vi "Dashboard Main.vi"() -> ()   [LabVIEW 2012]
uses:
  <vilib>/event_ctls.llb/eventvkey.ctl
  <vilib>/Utility/config.llb/NI_LVConfig.lvlib
  <vilib>/Utility/config.llb/Read Key (I32).vi
  <vilib>/Utility/config.llb/Write Key (I32).vi
  <vilib>/Utility/config.llb/Read Key (String).vi
  <vilib>/Utility/config.llb/Write Key (String).vi
  <vilib>/Rock Robotics/WPI/Camera/WPI_CameraFrameRate.ctl
  <vilib>/Rock Robotics/WPI/Camera/WPI_CameraExposure Values.ctl
  <vilib>/Rock Robotics/WPI/Camera/WPI_CameraWhite Balance Values.ctl
  <vilib>/Rock Robotics/WPI/Camera/WPI_CameraImageSize.ctl
panel:
  in  "Image Size":T1=enum."160x120"
  in  "Camera?":bool
  out "Battery Value":dbl(slide) scale=0.0..14.0 scale format="%#_2e"
  out "Battery":sgl(graph)
  in  "Camera Settings":T2={"Frate Rate"=30, "Compression"=30, "Size"=1} {"Frate Rate" scale=1.0..30.0; "Size" items=["640x480", "320x240", "160x120"]}
  out "Mode":T3(ring)=enum."Auto Disabled"
  out "Camera IP":string
  out "JS1 Z":dbl(slide) scale=-1.0..1.0 scale format="%#_2e"
  out "JS2 Z":dbl(slide) scale=-1.0..1.0 scale format="%#_2e"
  out "Joystick 1":cluster{"X":dbl, "Y":dbl}[](graph)
  out "Joystick 2":cluster{"X":dbl, "Y":dbl}[](graph)
  out "JS Buttons 1":T4
  out "JS Buttons 2":T4
  out "MotorSlide4":dbl(slide) scale=-1.0..1.0 scale format="%#_2e"
  out "MotorSlide3":dbl(slide) scale=-1.0..1.0 scale format="%#_2e"
  out "MotorSlide2":dbl(slide) scale=-1.0..1.0 scale format="%#_2e"
  in  "MotorName3":string="Front Left"
  in  "MotorName4":string="Front Right"
  in  "MotorName1":string="Rear Left"
  in  "MotorName2":string="Rear Right"
  out "MotorChart4":dbl(graph)
  out "MotorChart3":dbl(graph)
  out "MotorChart2":dbl(graph)
  out "MotorSlide1":dbl(slide) scale=-1.0..1.0 scale format="%#_2e"
  out "MotorChart1":dbl(graph)
  out "Robot IP":string
  in  "Dashboard Tab":enum32{"Operation", "Test", "Checklist"}(tab)
  in  "Checkbox 2":bool
  in  "Checkbox 1":bool
  in  "Slider 1":dbl(slide) scale=0.0..100.0
  in  "Slider":dbl(slide) scale=0.0..100.0 scale format="%#_3g"
  in  "On/Off":bool caption="Solenoid"
  in  "Test Name":u16(ring) items=["Select the test to run...", "Example Test", "-------------------------------", "List of tests is built in robot code.", "Replace with your own automated tests."]
  in  "Test Tree":string(tree)
  in  "Motor":cluster{"Value":dbl, "Enable":bool} {"Value" scale=-1.0..1.0 scale format="%#_3g"}
  out "Progress":T5 {"Test Progress" scale=0.0..100.0}
  in  "Rev/Fwd":cluster{"Forward":bool, "Reverse":bool}
  in  "Ring":u16(ring) items=["Auto", "Fixed indoor", "Fixed outdoor 1", "Fixed outdoor 2", "Fixed fluorescent 1", "Fixed fluorescent 2", "Hold current"]
  in  "Listbox":i32(listbox)
  in  "Viewer":T6(tab)
  out "Mbps":dbl format="%#.1g"
  in  "Enable":bool
  in  "DB Camera Config":bool
  out "Mbps":bool
  out "fps":dbl format="%#.1g"
  out "Image Error Message":string="Timeout in Camera Communications"
  out "Camera Image":T7(plugin-control)
  out "Tree":string(tree)
  # "Drive & Motors"
  # "Robot IP:"
  # "Customize by placing controls and indicators here and name to match\nDashboard Variables on robot."
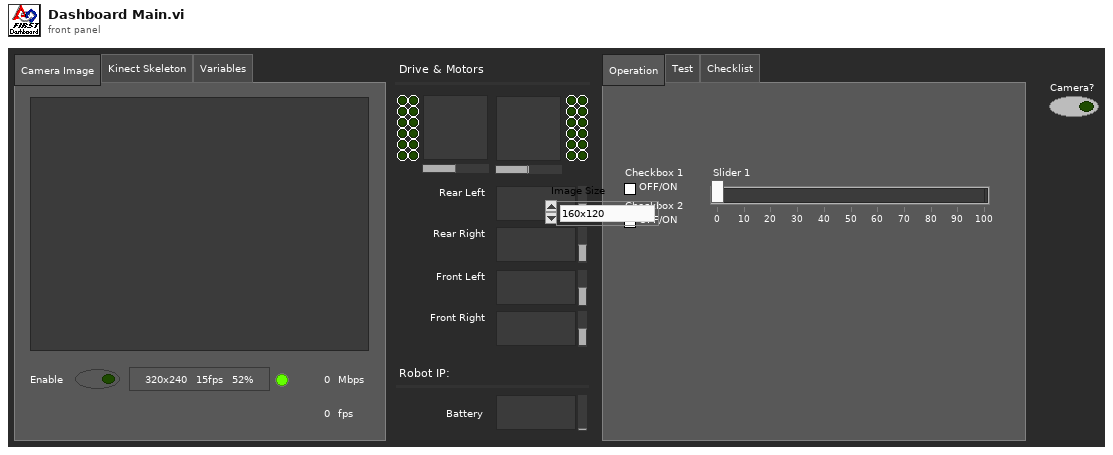
[diagram p1: front panel]
types:
  T1 = typedef "WPI_CameraImageSize.ctl" = enum16{"640x480", "320x240", "160x120"}
  T2 = cluster{"Frate Rate":i32, "Compression":i32, "Size":u16}
  T3 = enum8{"Tele-Op Disabled", "Tele-Op Enabled", "Auto Disabled", "Auto Enabled", "Test Disabled", "Test Enabled", ""}
  T4 = cluster{bool, bool, bool, bool, bool, bool, bool, bool, bool, bool, bool, bool}
  T5 = cluster{"Test Progress":u8, "Test Progress Text":string}
  T6 = enum32{"Camera Image", "Kinect Skeleton", "Variables"}
  T7 = typedef "IMAQ Image.ctl" = refnum<image>
  T8 = typedef "Image Type" = u32
  T9 = typedef "LVRectTypeDef.ctl" = cluster{"Left":i16, "Top":i16, "Right":i16, "Bottom":i16}
  T10 = typedef "WPI_CameraFrameRate.ctl" = u32
  T11 = typedef "WPI_CameraExposure Values.ctl" = enum16{"Auto", "Flicker-free 50 Hz", "Flicker-free 60 Hz", "Hold current"}
  T12 = typedef "WPI_CameraWhite Balance Values.ctl" = enum16{"Auto", "Fixed indoor", "Fixed outdoor 1", "Fixed outdoor 2", "Fixed fluorescent 1", "Fixed fluorescent 2", "Hold current"}
  T13 = typedef "WPI_CameraDevRef.ctl" = cluster{"Camera Address":string, "CameraStatus":errorcluster, "Acquire Image Notifier":refnum<notifier>}
  T14 = cluster{"Competition mode":bool, "Robot Link":bool, "Autonomous":bool, "Enabled":bool, "E-Stop":bool, "Simulated":bool, "TestMode":bool, "Docked Window":bool}
  T15 = cluster{"Boolean Array[0]":bool, "Boolean Array[1]":bool, "Boolean Array[2]":bool, "Boolean Array[3]":bool, "Boolean Array[4]":bool, "Boolean Array[5]":bool, "Boolean Array[6]":bool, "Boolean Array[7]":bool, "Boolean Array[8]":bool, "Boolean Array[9]":bool, "Boolean Array[10]":bool, "Boolean Array[11]":bool}
  T16 = typedef "NI_LVConfig.lvlib/Config Data RefNum.ctl" = refnum<k1>
  T17 = typedef "eventvkey.ctl" = enum16{"ASCII", "Enter", "Return", "Shift", "Ctrl", "Alt", "Cmd", "Opt", "Caps", "NumLock", "Clear", "Break", "Up", "Down", "Left", "Right", "Insert", "Delete", "Home", "End", "PageUp", "PageDown", "Escape", "Help", "Pause", "ScrollLock", "F1", "F2", "F3", "F4", "F5", "F6", "F7", "F8", "F9", "F10", "F11", "F12", "F13", "F14", "F15", "F16", "F17", "F18", "F19", "F20", "F21", "F22", "F23", "F24", "Play", "VolumeUp", "VolumeDown", "Mute", "Two Byte Char"}
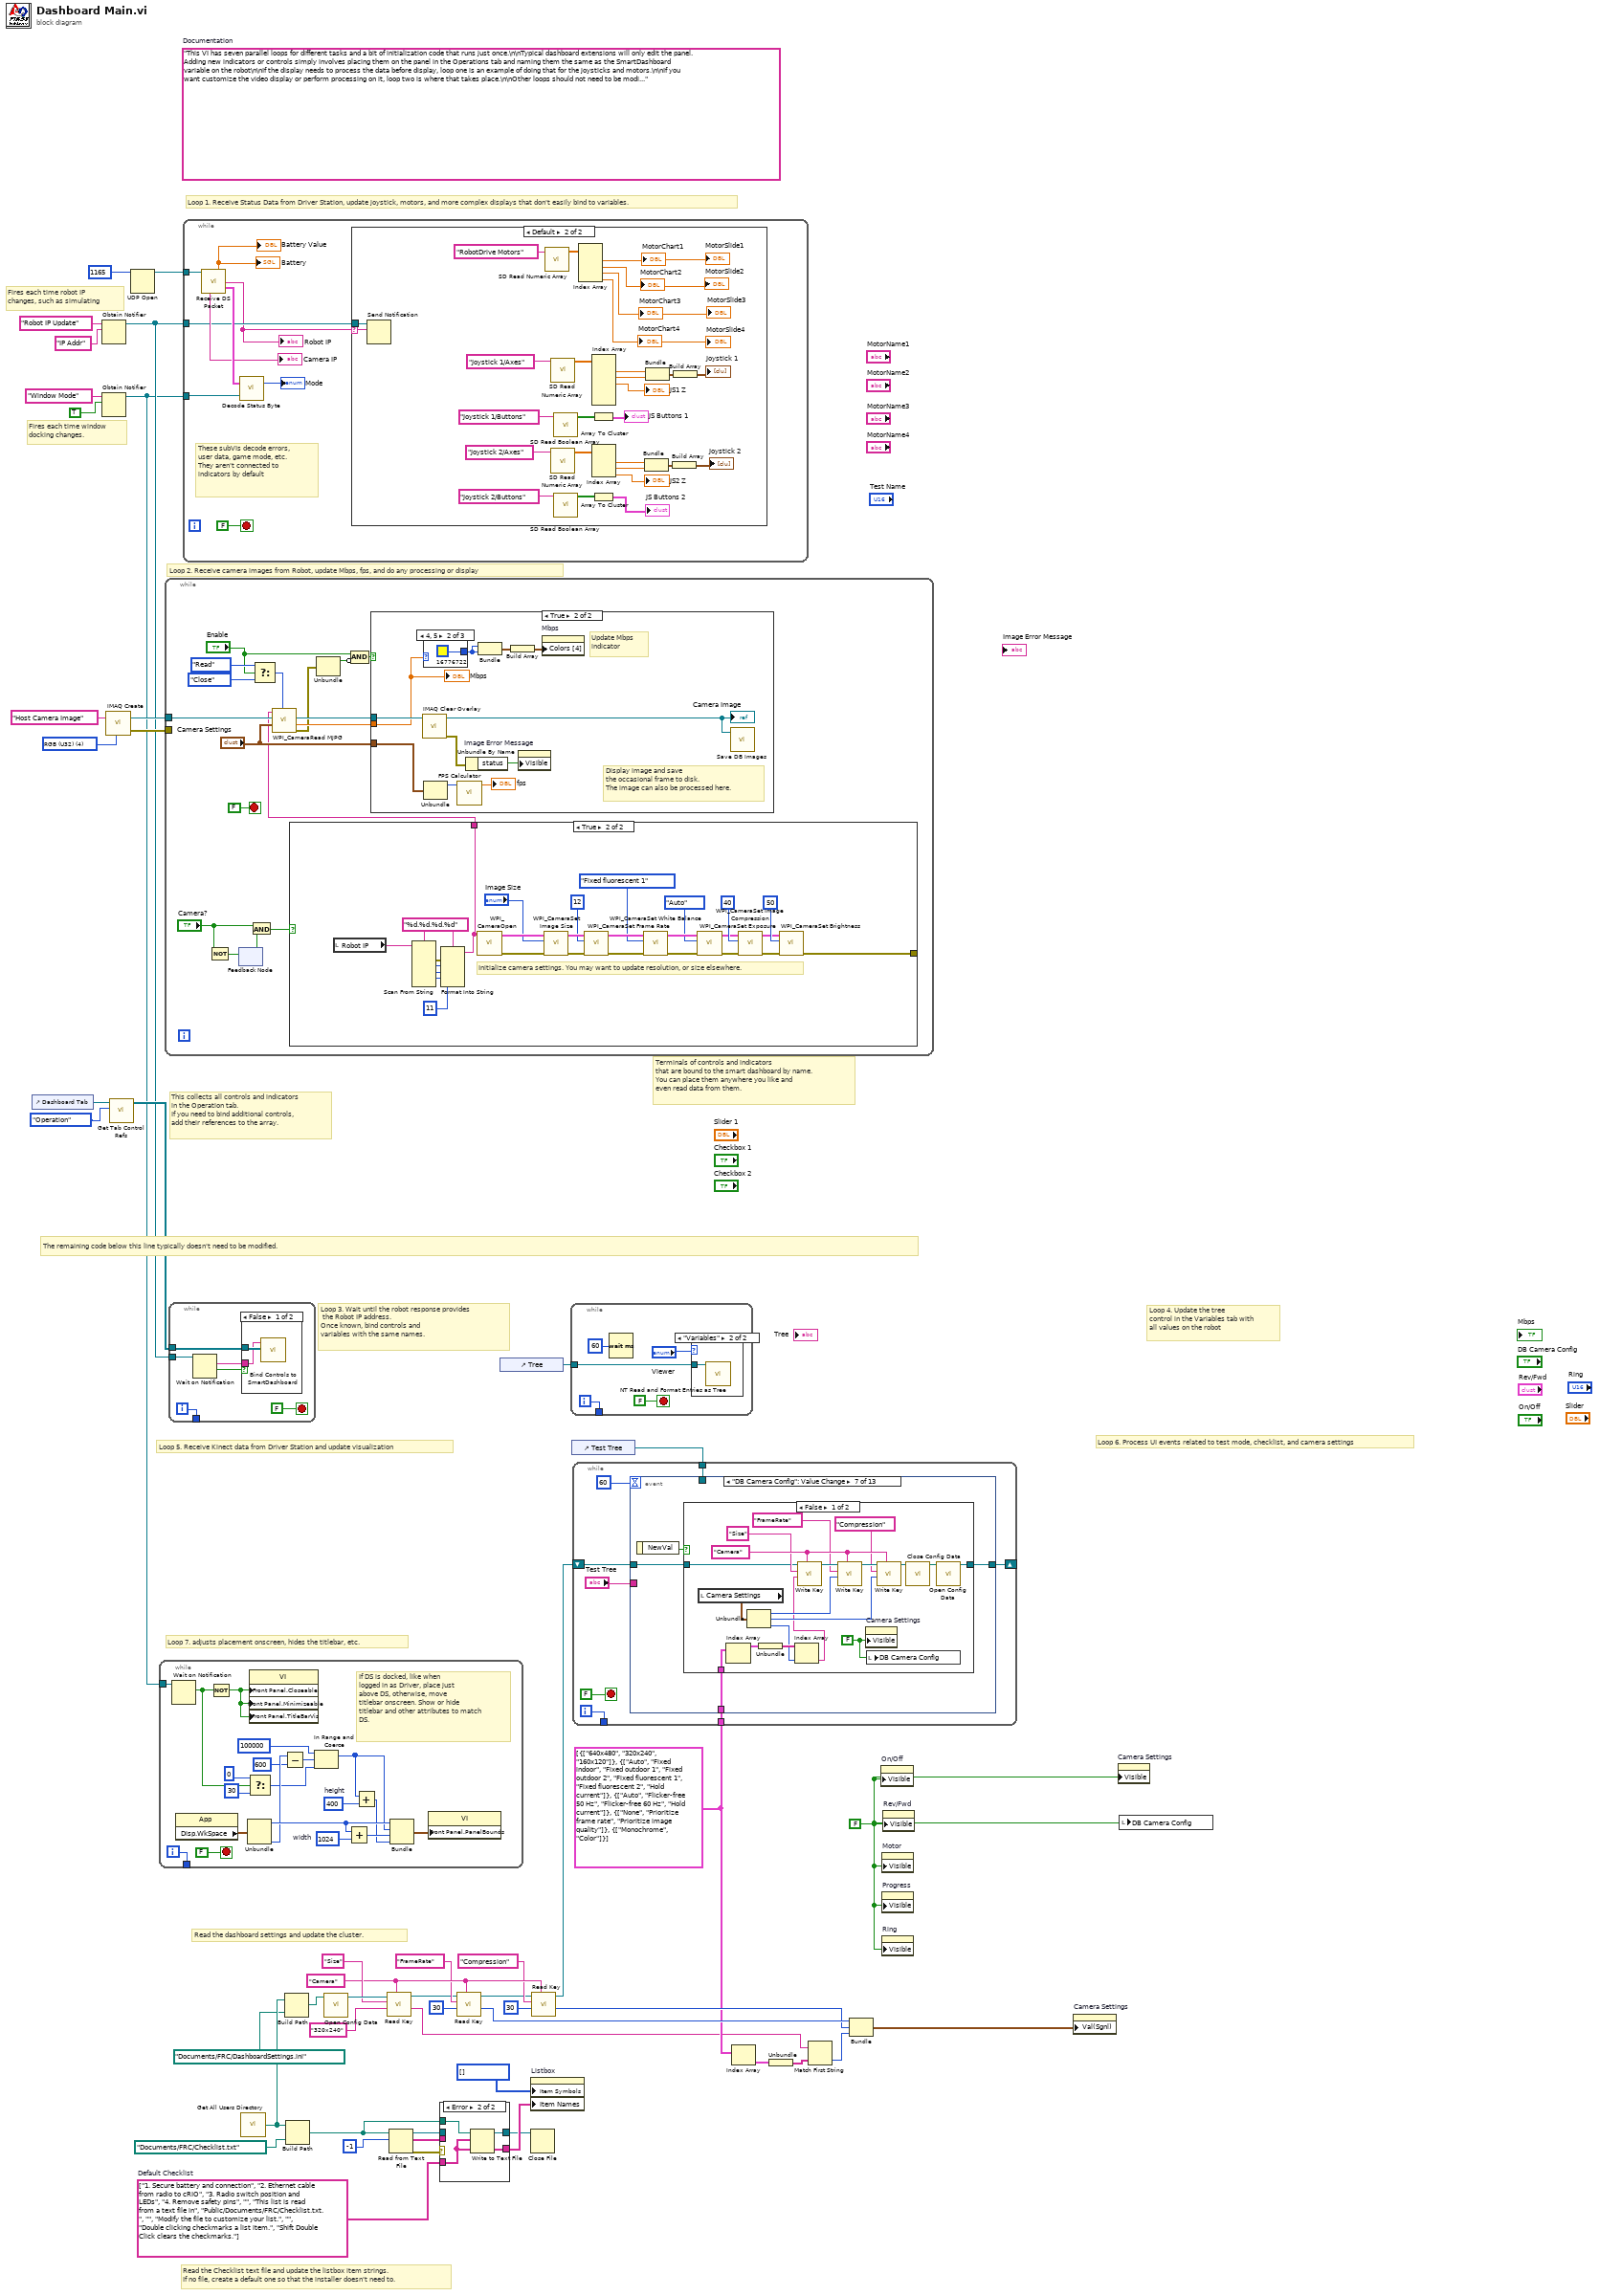
[diagram p0: block diagram]
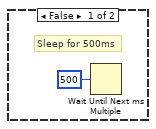
[diagram p4: hidden frame]
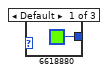
[diagram p5: hidden frame]
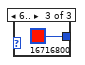
[diagram p6: hidden frame]
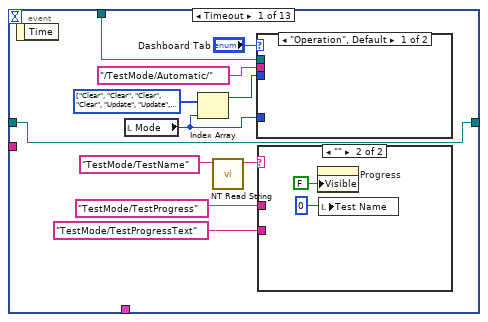
[diagram p8: hidden frame]
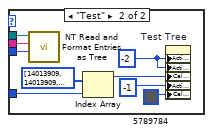
[diagram p9: hidden frame]
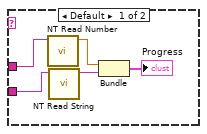
[diagram p10: hidden frame]
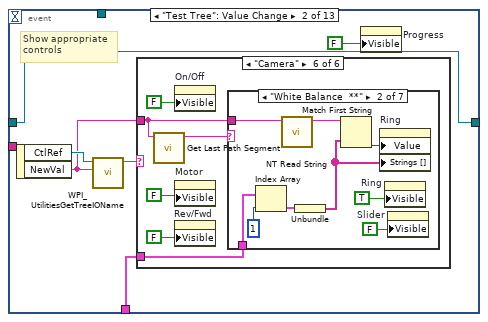
[diagram p11: hidden frame]
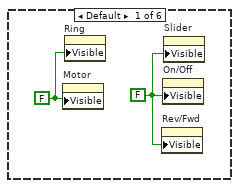
[diagram p12: hidden frame]
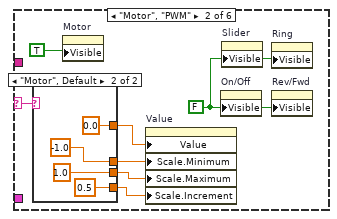
[diagram p13: hidden frame]
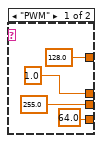
[diagram p14: hidden frame]
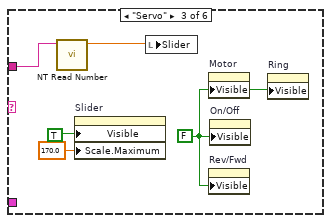
[diagram p15: hidden frame]
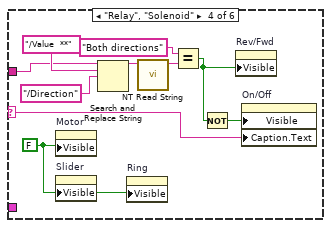
[diagram p16: hidden frame]
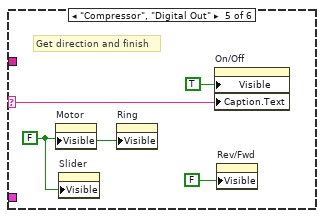
[diagram p17: hidden frame]
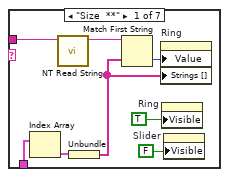
[diagram p18: hidden frame]
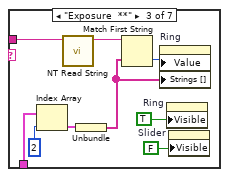
[diagram p19: hidden frame]
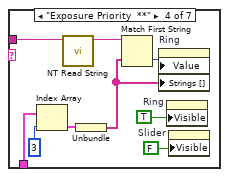
[diagram p20: hidden frame]
diagram:
  w21 = "Camera"
  w13 = cluster{string[]}[] [{["640x480", "320x240", "160x120"]}, {["Auto", "Fixed indoor", "Fixed outdoor 1", "Fixed outdoor 2", "Fixed fluorescent 1", "Fixed fluorescent 2", "Hold current"]}, {["Auto", "Flicker-free 50 Hz", "Flicker-free 60 Hz", "Hold current"]}, {["None", "Prioritize frame rate", "Prioritize image quality"]}, {["Monochrome", "Color"]}]
  w29 = string[] ["1. Secure battery and connection", "2. Ethernet cable from radio to cRIO", "3. Radio switch position and LEDs", "4. Remove safety pins", "", "This list is read from a text file in", "Public/Documents/FRC/Checklist.txt.", "", "Modify the file to customize your list.", "", "Double clicking checkmarks a list item.", "Shift Double Click clears the checkmarks."]  # Default Checklist
  w27 = FALSE ("Visible")
  (unwired) "This VI has seven parallel loops for different tasks and a bit of initialization code that runs just once.\n\nTypical dashboard extensions will only edit the panel. Adding new indicators or controls simply involves placing them on the panel in the Operations tab and naming them the same as the SmartDashboard variable on the robot\n\nIf the display needs to process the data before display, loop one is an example of doing that for the joysticks and motors.\n\nIf you want customize the video display or perform processing on it, loop two is where that takes place.\n\nOther loops should not need to be modified. They are pretty standard, and document the task they perform."  # Documentation
  w48 = T8 4 items=["Grayscale (U8)", "Grayscale (I16)", "Grayscale (SGL)", "Complex (CSG)", "RGB (U32)", "HSL (U32)", "RGB (U64)"] ("Image Type")
  # "Fires each time robot IP\nchanges, such as simulating"
  # "Fires each time window\ndocking changes."
  # "Read the Checklist text file and update the listbox item strings.\nIf no file, create a default one so that the installer doesn't need to."
  # "This collects all controls and indicators\nin the Operation tab.\nIf you need to bind additional controls,\nadd their references to the array."
  # "The remaining code below this line typically doesn't need to be modified."
  # "Loop 6. Process UI events related to test mode, checklist, and camera settings"
  # "Read the dashboard settings and update the cluster."
  # "Terminals of controls and indicators\nthat are bound to the smart dashboard by name.\nYou can place them anywhere you like and\neven read data from them."
  # "Loop 4. Update the tree\ncontrol in the Variables tab with\nall values on the robot"
  # "Loop 3. Wait until the robot response provides\n the Robot IP address.\nOnce known, bind controls and\nvariables with the same names."
  # "Loop 5. Receive Kinect data from Driver Station and update visualization"
  # "Loop 7. adjusts placement onscreen, hides the titlebar, etc."
  # "Loop 1. Receive Status Data from Driver Station, update joystick, motors, and more complex displays that don't easily bind to variables."
  # "Loop 2. Receive camera images from Robot, update Mbps, fps, and do any processing or display"
  n1 = control-ref of="Dashboard Tab"() -> (w43:refnum<vi>)
  n2 = Obtain Notifier(name (unnamed)="Robot IP Update", notification data type="IP Addr" ("name (unnamed)")) -> (notifier out=w40:refnum<notifier>)  [unwired: 2 in, 2 out]
  n3 = Obtain Notifier(name (unnamed)="Window Mode", notification data type=TRUE) -> (notifier out=w33:refnum<notifier>)  [unwired: 2 in, 2 out]
  n4 = call "IMAQ Create"("Image Name"="Host Camera Image", "Image Type"=w48) -> ("New Image"=w46:T7, "error out"=w45:errorcluster)  [unwired: 2 in, 1 out]
  n5 = call <vilib>:"Get Tab Control Refs.vi"("Page Index"=enum32{"Operation", "Test"}."Operation" ("Dashboard Tab"), "TabControl in"=w43) -> ("ControlsOnPage"=w44:refnum<vi>[])  [unwired: 9 in]
  n6 = UDP Open(11:u16 1165 ("port")) -> (port=w49:refnum<k16>)  [unwired: 2 in, 4 out]
  n7 = while {
    tunnel: w33 -> [w69]
    tunnel: [w67] -> _
    i -> [w67]
    stop <- FALSE stop-if-true
    w59 = 1024  # width
    w62 = 400  # height
    # "If DS is docked, like when\nlogged in as Driver, place just\nabove DS, otherwise, move\ntitlebar onscreen. Show or hide\ntitlebar and other attributes to match\nDS."
    n8 = Wait on Notification(notifier=w69) -> (notification=w54:bool)  [unwired: 3 in, 3 out]
    n9 = property class="App"() -> ("Disp.WkSpace"=w65:T9)  [unwired: 2 in, 2 out]
    n10 = Not(x=w54) -> (.not. x?=w68:bool)
    n11 = Unbundle(w65) -> ("Left"=w63:i16, "Bottom"=w60:i16)  [unwired: 2 out]
    n12 = Select(t=0, s=w54, f=30) -> (s? t:f=w53:i32)
    n13 = property class="VI"("Front Panel.Closeable"=w68, "Front Panel.Minimizeable"=w68, "Front Panel.TitleBarVis"=w68) -> ()  [unwired: 2 in, 2 out]
    n14 = Subtract(x=w60, y=600) -> (x-y=w57:i32)
    n15 = In Range and Coerce(upper limit=100000, x=w57, lower limit=w53) -> (coerced(x)=w51:i32)  [unwired: 1 out]
    n16 = Add(x=w63, y=w59) -> (x+y=w64:i32)
    n17 = Add(x=w51, y=w62) -> (x+y=w61:i32)
    n18 = Bundle("Left"=w63, w51, w64, w61) -> (w66:cluster{"Left":i16, i32, i32, i32})  [unwired: 1 out]
    n19 = property class="VI"("Front Panel.PanelBounds"=w66) -> ()  [unwired: 2 in, 2 out]
  }
  n20 = while {
    tunnel: w46 -> [w85]
    tunnel: w45 -> [_]
    stop <- FALSE stop-if-true
    n21 = Not(x="Camera?") -> (.not. x?=w75:bool)
    n22 = feedback #1() -> (w74:bool)  [unwired: 1 in]
    n23 = feedback-in #1(w75) -> ()
    n24 = And(x="Camera?", y=w74) -> (x .and. y?=w72:bool)
    n25 = Select(t=enum16{"Read", "Reopen", "Close"}."Read" ("Operation"), s="Enable", f=enum16{"Read", "Reopen", "Close"}."Close" ("Operation")) -> (s? t:f=w80:enum16{"Read", "Reopen", "Close"})
    n26 = case shown="True" w72 {
      tunnel: [_ w89] -> _
      tunnel: [_ w88] -> w71
      frame False {
      }
      frame True {
        w96 = "%d.%d.%d.%d" ("format string")
        # "Initialize camera settings. You may want to update resolution, or size elsewhere."
        n27 = local read "Robot IP"() -> (w90:string)
        n28 = Scan From String(format string=w96, input string=w90) -> (error out=w94:errorcluster, output 1=w93:i32, output 2=w92:i32, output 3=w91:i32)  [unwired: 2 in, 7 out]
        n29 = Format Into String(format string=w96, error in=w94, w93, w92, w91, 11 ("IP Suffix:")) -> (resulting string=w88:string)  [unwired: 1 in, 1 out]
        n30 = call <vilib>:"WPI_CameraOpen.vi"("Camera Address"=w88) -> ("error out"=w106:errorcluster, "CameraDevRef"=w107:T13)  [unwired: 2 in, 7 out]
        n31 = call <vilib>:"WPI_CameraSet Image Size.vi"("error in (no error)"=w106, "Image Size"="Image Size", "CameraDevRef"=w107) -> ("error out"=w105:errorcluster, "CameraDevRef Out"=w108:T13)  [unwired: 7 out]
        n32 = call <vilib>:"WPI_CameraSet Frame Rate.vi"("error in (no error)"=w105, "Frame Rate (fps)"=T10 12, "CameraDevRef"=w108) -> ("error out"=w104:errorcluster, "CameraDevRef Out"=w110:T13)  [unwired: 7 out]
        n33 = call <vilib>:"WPI_CameraSet White Balance.vi"("error in (no error)"=w104, "White Balance"=WPI_CameraWhite_Balance_Values."Fixed fluorescent 1", "CameraDevRef"=w110) -> ("error out"=w103:errorcluster, "CameraDevRef Out"=w109:T13)  [unwired: 7 out]
        n34 = call <vilib>:"WPI_CameraSet Exposure.vi"("error in (no error)"=w103, "Exposure"=WPI_CameraExposure_Values."Auto", "CameraDevRef"=w109) -> ("error out"=w102:errorcluster, "CameraDevRef Out"=w112:T13)  [unwired: 7 out]
        n35 = call <vilib>:"WPI_CameraSet Image Compression.vi"("error in (no error)"=w102, "Compression"=40, "CameraDevRef"=w112) -> ("error out"=w101:errorcluster, "CameraDevRef Out"=w111:T13)  [unwired: 7 out]
        n36 = call <vilib>:"WPI_CameraSet Brightness.vi"("error in (no error)"=w101, "Brightness"=50, "CameraDevRef"=w111) -> ("error out"=w89:errorcluster)  [unwired: 8 out]
      }
    }
    n37 = call <vilib>:"WPI_CameraRead MJPG.vi"("Operation"=w80, "Camera Settings"="Camera Settings", "Image"=w85, "address"=w71) -> ("error out"=w79:errorcluster, "Bandwidth (kbps)"=w83:dbl, "Image Out"=w84:T7)  [unwired: 5 in]
    n38 = Unbundle(w79) -> ("status"=w77:bool)  [unwired: 2 out]
    n39 = Compound Arithmetic op=AND("Enable", invert w77) -> (w76:bool)
    n40 = case shown="True" w76 {
      tunnel: "Camera Settings" -> [_ w117]
      tunnel: w84 -> [_ w120]
      tunnel: w83 -> [_ w119]
      frame False {
        # "Sleep for 500ms"
        n41 = Wait Until Next ms Multiple(millisecond multiple=u32 500) -> ()  [unwired: 1 out]
      }
      frame True {
        # "Display image and save\nthe occasional frame to disk.\nThe image can also be processed here."
        # "Update Mbps\nindicator"
        n42 = call "IMAQ Clear Overlay"("Image"=w120) -> ("error out"=w125:errorcluster, "Image Out"=w124:T7)  [unwired: 2 in, 7 out]
        "Camera Image" <- w124
        n43 = case shown="4, 5" w119 {
          tunnel: [u32 6618880 ("Color Box") u32 16776722 ("Color Box") u32 16716800 ("Color Box")] -> w121
          frame Default {
          }
          frame 4, 5 {
          }
          frame 6.. {
          }
        }
        n44 = Unbundle(w117) -> ("Frate Rate"=w116:i32)  [unwired: 2 out]
        n45 = call "FPS Calculator.vi"("Average Count"=w116) -> ("fps"=→"fps":dbl)  [unwired: 10 in]
        n46 = Unbundle By Name(w125) -> ("status"=w126:bool)
        n47 = Bundle("Color Box"=w121, "Color Box"=w121) -> (w123:cluster{"Color Box":u32, "Color Box":u32})  [unwired: 1 out]
        n48 = Build Array(w123) -> (w122:cluster{"Color Box":u32, "Color Box":u32}[])
        n49 = property on="Image Error Message" class="Str"("Visible"=w126) -> ()  [unwired: 2 in, 2 out]
        n50 = property on="Mbps" class="Bool (strict)"("Colors [4]"=w122) -> ()  [unwired: 2 in, 2 out]
        n51 = call "Save DB Images.vi"("Image"=w124) -> ()  [unwired: 2 in, 1 out]
        "Mbps" <- w119
      }
    }
  }
  n52 = while {
    tunnel: w44 -> [w135]
    tunnel: w40 -> [w132]
    tunnel: [w130] -> _
    i -> [w130]
    stop <- FALSE stop-if-true
    n53 = Wait on Notification(notifier=w132) -> (notification=w131:string, timed out?=w133:bool)  [unwired: 3 in, 2 out]
    n54 = case shown="False" w133 {
      tunnel: w135 -> [w137 _]
      tunnel: w131 -> [w136 _]
      frame False {
        n55 = call <vilib>:"Bind Controls to SmartDashboard.vi"("Bound Control Refs"=w137, "Server IP Address"=w136) -> ()  [unwired: 10 in]
      }
      frame True {
      }
    }
  }
  n56 = while {
    tunnel: w49 -> [w144]
    tunnel: w40 -> [w139]
    tunnel: w33 -> [w142]
    stop <- FALSE stop-if-true
    # "These subVIs decode errors, user data, game mode, etc.\nThey aren't connected to indicators by default"
    n57 = call "Receive DS Packet.vi"("Recv Socket"=w144) -> ("Battery"=→"Battery" →"Battery Value":sgl, "Robot IP Address"=w138:string, "Status"=w145:T14, "Camera IP Address"=→"Camera IP":string)  [unwired: 1 in, 10 out]
    "Robot IP" <- w138
    n58 = call "Decode Status Byte.vi"("Window Mode Notifier"=w142, "Status"=w145) -> ("Mode"=→"Mode":T3)  [unwired: 1 out]
    n59 = case shown="Default" w138 {
      selector: w138 -> [_ w147]
      tunnel: w139 -> [_ w148]
      frame "0.0.0.0" {
        # "Robot not responding, don't poll the variables"
      }
      frame Default {
        n60 = Send Notification(notification=w147, notifier=w148) -> ()  [unwired: 1 in, 2 out]
        n61 = call <vilib>:"SD Read Numeric Array.vi"("Name"="RobotDrive Motors") -> ("Numeric Array"=w171:dbl[])  [unwired: 8 in, 2 out]
        n62 = call <vilib>:"SD Read Numeric Array.vi"("Name"="Joystick 1/Axes") -> ("Numeric Array"=w164:dbl[])  [unwired: 8 in, 2 out]
        n63 = call <vilib>:"SD Read Numeric Array.vi"("Name"="Joystick 2/Axes") -> ("Numeric Array"=w158:dbl[])  [unwired: 8 in, 2 out]
        n64 = call <vilib>:"SD Read Boolean Array.vi"("Name"="Joystick 1/Buttons") -> ("Boolean Array"=w166:bool[])  [unwired: 8 in, 2 out]
        n65 = call <vilib>:"SD Read Boolean Array.vi"("Name"="Joystick 2/Buttons") -> ("Boolean Array"=w157:bool[])  [unwired: 8 in, 2 out]
        n66 = Index Array(array=w171) -> (element #1=→"MotorChart1" →"MotorSlide1":dbl, element #2=→"MotorSlide2" →"MotorChart2":dbl, element #3=→"MotorChart3" →"MotorSlide3":dbl, element #4=→"MotorChart4" →"MotorSlide4":dbl)  [unwired: 4 in]
        n67 = Array To Cluster(array=w166) -> (cluster=→"JS Buttons 1":T15)
        n68 = Array To Cluster(array=w157) -> (cluster=→"JS Buttons 2":T15)
        n69 = Index Array(array=w164) -> (element #1=w161:dbl, element #2=w162:dbl, element #3=→"JS1 Z":dbl)  [unwired: 6 in, 3 out]
        n70 = Index Array(array=w158) -> (element #1=w153:dbl, element #2=w152:dbl, element #3=→"JS2 Z":dbl)  [unwired: 3 in]
        n71 = Bundle("Numeric"=w153, "Numeric"=w152) -> (w154:cluster{"Numeric":dbl, "Numeric":dbl})  [unwired: 1 in]
        n72 = Bundle("Numeric"=w161, "Numeric"=w162) -> (w160:cluster{"Numeric":dbl, "Numeric":dbl})  [unwired: 1 in]
        n73 = Build Array(w154) -> (→"Joystick 2":cluster{"Numeric":dbl, "Numeric":dbl}[])
        n74 = Build Array(w160) -> (→"Joystick 1":cluster{"Numeric":dbl, "Numeric":dbl}[])
      }
    }
  }
  n75 = call "Get All Users Directory.vi"() -> ("All User Path"=w26:path)
  n76 = Build Path(base path=w26, name or relative path=path "Documents/FRC/DashboardSettings.ini") -> (appended path=w25:path)
  n77 = Build Path(base path=w26, name or relative path=path "Documents/FRC/Checklist.txt") -> (appended path=w30:path)
  n78 = call <vilib>:"Open Config Data.vi"("configuration file path"=w25) -> ("refnum"=w24:T16)  [unwired: 8 in, 2 out]
  n79 = call-poly <vilib>:"Read Key.vi"("section"=w21, "default value"="320x240", "key"="Size", "refnum"=w24) -> ("value"=w11:string, "refnum out"=w6:T16)  [unwired: 2 in, 4 out]
  n80 = Read from Text File(file (use dialog)=w30, count=-1 ("timeout ms (25000)")) -> (refnum out=w8:refnum<file>, text=w31:string[], error out=w32:errorcluster)  [unwired: 2 in, 1 out]
  n81 = case shown="Error" w32 {
    tunnel: w31 -> [w176 _]
    tunnel: [w176 w178] -> w28
    tunnel: w29 -> [_ w178]
    tunnel: w30 -> [_ w179]
    tunnel: [w175 w177] -> w7
    tunnel: w8 -> [w175 _]
    frame No Error {
    }
    frame Error {
      n82 = Write to Text File(file (use dialog)=w179, text=w178) -> (refnum out=w177:refnum<file>)  [unwired: 2 in, 2 out]
    }
  }
  n83 = call-poly <vilib>:"Read Key.vi"("section"=w21, "default value"=30, "key"="FrameRate", "refnum"=w6) -> ("value"=w16:i32, "refnum out"=w5:T16)  [unwired: 1 in, 5 out]
  n84 = control-ref of="Tree"() -> (w2:refnum<vi>)
  n85 = property on="Listbox" class="LstBox (strict)"("Item Symbols"=i32[] [], "Item Names"=w28) -> ()  [unwired: 2 in, 2 out]
  n86 = Close File(refnum=w7) -> ()  [unwired: 1 in, 2 out]
  n87 = call-poly <vilib>:"Read Key.vi"("section"=w21, "default value"=30, "key"="Compression", "refnum"=w5) -> ("value"=w15:i32, "refnum out"=w3:T16)  [unwired: 1 in, 5 out]
  n88 = while {
    tunnel: [w181] -> _
    tunnel: w2 -> [w180]
    i -> [w181]
    stop <- FALSE stop-if-true
    n89 = Wait (ms)(milliseconds to wait=u32 60) -> ()  [unwired: 1 out]
    n90 = case shown="\"Variables\"" "Viewer" {
      tunnel: w180 -> [_ w185]
      frame Default {
      }
      frame "Variables" {
        n91 = call <vilib>:"NT Read and Format Entries as Tree.vi"("Tree Refnum"=w185) -> ()  [unwired: 9 in, 2 out]
      }
    }
  }
  n92 = control-ref of="Test Tree"() -> (w1:refnum<vi>)
  n93 = while {
    tunnel: w13 -> [w190]
    shift-right: [w189] -> _
    shift-left: w3 -> [w188]
    tunnel: [w187] -> _
    tunnel: w1 -> [w186]
    i -> [w187]
    stop <- FALSE stop-if-true
    n94 = event shown="[6] \"DB Camera Config\": Value Change" {
      selector: _ -> [_ _ _ _ _ _ _ _ _ _ _ _ _]
      dyn-events: _ -> [_ _ _ _ _ _ _ _ _ _ _ _ _]
      timeout: u32 60 ("milliseconds to wait") -> [_ _ _ _ _ _ _ _ _ _ _ _ _]
      tunnel: w186 -> [w200 _ _ _ _ _ _ _ _ _ _ _ _]
      tunnel: "Test Tree" -> [_ _ _ _ _ _ _ _ w394 w402 w404 w408 w416]
      tunnel: w190 -> [_ w222 _ _ _ _ w358 w388 _ _ _ _ _]
      tunnel: [w194 w221 _ w324 w332 w344 w357 w381 w393 w400 w403 w407 w415] -> w189
      tunnel: w188 -> [w194 w221 _ w324 w332 w344 w356 w381 w393 w400 w403 w407 w415]
      event Timeout {
        w199 = enum16{"Update", "Clear"}[] [enum."Clear", enum."Clear", enum."Clear", enum."Clear", enum."Update", enum."Update", enum."Clear"] items=["Update", "Clear"]
        n95 = event-data() -> ()  [unwired: 1 in, 1 out]
        n96 = local read "Mode"() -> (w197:T3)
        n97 = Index Array(array=w199, index=w197) -> (element=w198:enum16{"Update", "Clear"})
        n98 = call <vilib>:"NT Read String.vi"("Name"="TestMode/TestName") -> ("String"=w203:string)  [unwired: 9 in, 1 out]
        n99 = case shown="\"Operation\", Default" "Dashboard Tab" {
          tunnel: w200 -> [_ w213]
          tunnel: "/TestMode/Automatic/" ("Name Pattern") -> [_ w212]
          tunnel: w198 -> [_ w211]
          tunnel: w197 -> [_ w209]
          frame "Operation", Default {
          }
          frame "Test" {
            w208 = -2 ("Active Item:Row Number")
            n100 = call <vilib>:"NT Read and Format Entries as Tree.vi"("Operation"=w211, "Name Pattern"=w212, "Tree Refnum"=w213) -> ()  [unwired: 7 in, 2 out]
            n101 = Index Array(array=u32[] [14013909, 14013909, 14013909, 14013909, 14013909, 16777215, 14013909], index=w209) -> (element=w207:u32)
            n102 = property on="Test Tree" class="Tree (strict)"("Active Item Row Number"=w208, "ActiveColNum"=w208, "CellBG"=w207, "Active Item Row Number"=-1 ("Active Item:Row Number"), "CellBG"=u32 5789784 ("Color Box")) -> ()  [unwired: 2 in, 2 out]
          }
        }
        n103 = case shown="\"\"" w203 {
          tunnel: "TestMode/TestProgress" ("Name") -> [w215 _]
          tunnel: "TestMode/TestProgressText" ("Name") -> [w214 _]
          frame Default {
            n104 = call <vilib>:"NT Read Number.vi"("Name"=w215) -> ("Numeric"=w216:dbl)  [unwired: 9 in, 1 out]
            n105 = call <vilib>:"NT Read String.vi"("Name"=w214) -> ("String"=w217:string)  [unwired: 9 in, 1 out]
            n106 = Bundle("Numeric"=w216, "String"=w217) -> (→"Progress":cluster{"Numeric":dbl, "String":string})  [unwired: 1 in]
          }
          frame "" {
            n107 = property on="Progress" class="Clust (strict)"("Visible"=FALSE) -> ()  [unwired: 2 in, 2 out]
            n108 = local write "Test Name"(u16 0) -> ()
          }
        }
      }
      event "Test Tree": Value Change {
        # "Show appropriate\ncontrols"
        n109 = event-data() -> ("CtlRef"=w225:refnum<vi>, "NewVal"=w223:string)  [unwired: 1 in]
        n110 = call <vilib>:"WPI_UtilitiesGetTreeIOName.vi"("NewVal"=w223, "TreeControl in"=w225) -> ("I/O Name"=w226:string)  [unwired: 9 in]
        n111 = case shown="\"Camera\"" w226 {
          selector: w226 -> [_ w233 _ w251 w260 _]
          tunnel: w223 -> [_ _ w248 w250 _ w267]
          tunnel: w222 -> [_ _ _ _ _ w266]
          frame Default {
            w228 = FALSE ("Visible")
            w227 = FALSE ("Visible")
            n112 = property on="Motor" class="Clust (strict)"("Visible"=w227) -> ()  [unwired: 2 in, 2 out]
            n113 = property on="Ring" class="Ring (strict)"("Visible"=w227) -> ()  [unwired: 2 in, 2 out]
            n114 = property on="Rev/Fwd" class="Clust (strict)"("Visible"=w228) -> ()  [unwired: 2 in, 2 out]
            n115 = property on="On/Off" class="Bool (strict)"("Visible"=w228) -> ()  [unwired: 2 in, 2 out]
            n116 = property on="Slider" class="Slide (strict)"("Visible"=w228) -> ()  [unwired: 2 in, 2 out]
          }
          frame "Motor", "PWM" {
            w234 = FALSE ("Visible")
            n117 = case shown="\"Motor\", Default" w233 {
              tunnel: [1.0 ("Value") -1.0 ("Value")] -> w232
              tunnel: [255.0 ("Value") 1.0 ("Value")] -> w231
              tunnel: [128.0 ("Value") 0.0 ("Value")] -> w230
              tunnel: [64.0 ("Value") 0.5 ("Value")] -> w229
              frame "PWM" {
              }
              frame "Motor", Default {
              }
            }
            n118 = property on="Motor" class="Clust (strict)"("Visible"=TRUE) -> ()  [unwired: 2 in, 2 out]
            n119 = property on="Value" class="Slide (strict)"("Value"=w230, "Scale.Minimum"=w232, "Scale.Maximum"=w231, "Scale.Increment"=w229) -> ()  [unwired: 2 in, 2 out]
            n120 = property on="On/Off" class="Bool (strict)"("Visible"=w234) -> ()  [unwired: 2 in, 2 out]
            n121 = property on="Slider" class="Slide (strict)"("Visible"=w234) -> ()  [unwired: 2 in, 2 out]
            n122 = property on="Ring" class="Ring (strict)"("Visible"=w234) -> ()  [unwired: 2 in, 2 out]
            n123 = property on="Rev/Fwd" class="Clust (strict)"("Visible"=w234) -> ()  [unwired: 2 in, 2 out]
          }
          frame "Servo" {
            w246 = FALSE ("Visible")
            n124 = call <vilib>:"NT Read Number.vi"("Name"=w248) -> ("Numeric"=w247:dbl)  [unwired: 9 in, 1 out]
            n125 = property on="Slider" class="Slide (strict)"("Visible"=TRUE, "Scale.Maximum"=170.0 ("Scale.Range:Maximum")) -> ()  [unwired: 2 in, 2 out]
            n126 = local write "Slider"(w247) -> ()
            n127 = property on="Motor" class="Clust (strict)"("Visible"=w246) -> ()  [unwired: 2 in, 2 out]
            n128 = property on="Rev/Fwd" class="Clust (strict)"("Visible"=w246) -> ()  [unwired: 2 in, 2 out]
            n129 = property on="On/Off" class="Bool (strict)"("Visible"=w246) -> ()  [unwired: 2 in, 2 out]
            n130 = property on="Ring" class="Ring (strict)"("Visible"=w246) -> ()  [unwired: 2 in, 2 out]
          }
          frame "Relay", "Solenoid" {
            w249 = FALSE ("Visible")
            n131 = property on="Motor" class="Clust (strict)"("Visible"=w249) -> ()  [unwired: 2 in, 2 out]
            n132 = property on="Slider" class="Slide (strict)"("Visible"=w249) -> ()  [unwired: 2 in, 2 out]
            n133 = Search and Replace String(input string=w250, search string="/Value  **", replace string="/Direction") -> (result string=w256:string)  [unwired: 5 in, 3 out]
            n134 = property on="Ring" class="Ring (strict)"("Visible"=w249) -> ()  [unwired: 2 in, 2 out]
            n135 = call <vilib>:"NT Read String.vi"("Name"=w256) -> ("String"=w254:string)  [unwired: 9 in, 1 out]
            n136 = Equal?(x="Both directions", y=w254) -> (x = y?=w252:bool)
            n137 = Not(x=w252) -> (.not. x?=w253:bool)
            n138 = property on="Rev/Fwd" class="Clust (strict)"("Visible"=w252) -> ()  [unwired: 2 in, 2 out]
            n139 = property on="On/Off" class="Bool (strict)"("Visible"=w253, "Caption.Text"=w251) -> ()  [unwired: 2 in, 2 out]
          }
          frame "Compressor", "Digital Out" {
            w259 = FALSE ("Visible")
            # "Get direction and finish"
            n140 = property on="Motor" class="Clust (strict)"("Visible"=w259) -> ()  [unwired: 2 in, 2 out]
            n141 = property on="Slider" class="Slide (strict)"("Visible"=w259) -> ()  [unwired: 2 in, 2 out]
            n142 = property on="Ring" class="Ring (strict)"("Visible"=w259) -> ()  [unwired: 2 in, 2 out]
            n143 = property on="On/Off" class="Bool (strict)"("Visible"=TRUE, "Caption.Text"=w260) -> ()  [unwired: 2 in, 2 out]
            n144 = property on="Rev/Fwd" class="Clust (strict)"("Visible"=FALSE) -> ()  [unwired: 2 in, 2 out]
          }
          frame "Camera" {
            n145 = call <vilib>:"Get Last Path Segment.vi"("String in"=w267) -> ("String out"=w268:string)  [unwired: 10 in]
            n146 = property on="On/Off" class="Bool (strict)"("Visible"=FALSE) -> ()  [unwired: 2 in, 2 out]
            n147 = property on="Motor" class="Clust (strict)"("Visible"=FALSE) -> ()  [unwired: 2 in, 2 out]
            n148 = property on="Rev/Fwd" class="Clust (strict)"("Visible"=FALSE) -> ()  [unwired: 2 in, 2 out]
            n149 = case shown="\"White Balance  **\"" w268 {
              tunnel: w267 -> [w274 w283 w292 w301 w310 _ w316]
              tunnel: w266 -> [w272 w280 w289 w298 w307 _ _]
              frame "Size  **" {
                n150 = Index Array(array=w272) -> (element=w271:cluster{string[]})  [unwired: 1 in]
                n151 = call <vilib>:"NT Read String.vi"("Name"=w274) -> ("String"=w273:string)  [unwired: 9 in, 1 out]
                n152 = Unbundle(w271) -> (w269:string[])
                n153 = Match First String(2:w269, 3:w273) -> (0:w270:i32)  [unwired: 1 out]
                n154 = property on="Ring" class="Ring (strict)"("Value"=w270, "Strings []"=w269) -> ()  [unwired: 2 in, 2 out]
                n155 = property on="Ring" class="Ring (strict)"("Visible"=TRUE) -> ()  [unwired: 2 in, 2 out]
                n156 = property on="Slider" class="Slide (strict)"("Visible"=FALSE) -> ()  [unwired: 2 in, 2 out]
              }
              frame "White Balance  **" {
                n157 = Index Array(array=w280, index=1) -> (element=w281:cluster{string[]})
                n158 = call <vilib>:"NT Read String.vi"("Name"=w283) -> ("String"=w282:string)  [unwired: 9 in, 1 out]
                n159 = Unbundle(w281) -> (w278:string[])
                n160 = Match First String(2:w278, 3:w282) -> (0:w277:i32)  [unwired: 1 out]
                n161 = property on="Ring" class="Ring (strict)"("Value"=w277, "Strings []"=w278) -> ()  [unwired: 2 in, 2 out]
                n162 = property on="Ring" class="Ring (strict)"("Visible"=TRUE) -> ()  [unwired: 2 in, 2 out]
                n163 = property on="Slider" class="Slide (strict)"("Visible"=FALSE) -> ()  [unwired: 2 in, 2 out]
              }
              frame "Exposure  **" {
                n164 = Index Array(array=w289, index=2) -> (element=w290:cluster{string[]})
                n165 = call <vilib>:"NT Read String.vi"("Name"=w292) -> ("String"=w291:string)  [unwired: 9 in, 1 out]
                n166 = Unbundle(w290) -> (w286:string[])
                n167 = Match First String(2:w286, 3:w291) -> (0:w287:i32)  [unwired: 1 out]
                n168 = property on="Ring" class="Ring (strict)"("Value"=w287, "Strings []"=w286) -> ()  [unwired: 2 in, 2 out]
                n169 = property on="Ring" class="Ring (strict)"("Visible"=TRUE) -> ()  [unwired: 2 in, 2 out]
                n170 = property on="Slider" class="Slide (strict)"("Visible"=FALSE) -> ()  [unwired: 2 in, 2 out]
              }
              frame "Exposure Priority  **" {
                n171 = Index Array(array=w298, index=3) -> (element=w299:cluster{string[]})
                n172 = call <vilib>:"NT Read String.vi"("Name"=w301) -> ("String"=w300:string)  [unwired: 9 in, 1 out]
                n173 = Unbundle(w299) -> (w295:string[])
                n174 = Match First String(2:w295, 3:w300) -> (0:w296:i32)  [unwired: 1 out]
                n175 = property on="Ring" class="Ring (strict)"("Value"=w296, "Strings []"=w295) -> ()  [unwired: 2 in, 2 out]
                n176 = property on="Ring" class="Ring (strict)"("Visible"=TRUE) -> ()  [unwired: 2 in, 2 out]
                n177 = property on="Slider" class="Slide (strict)"("Visible"=FALSE) -> ()  [unwired: 2 in, 2 out]
              }
              frame "Color Enable  **" {
                n178 = Index Array(array=w307, index=4) -> (element=w308:cluster{string[]})
                n179 = call <vilib>:"NT Read String.vi"("Name"=w310) -> ("String"=w309:string)  [unwired: 9 in, 1 out]
                n180 = Unbundle(w308) -> (w304:string[])
                n181 = Match First String(2:w304, 3:w309) -> (0:w305:i32)  [unwired: 1 out]
                n182 = property on="Ring" class="Ring (strict)"("Value"=w305, "Strings []"=w304) -> ()  [unwired: 2 in, 2 out]
                n183 = property on="Ring" class="Ring (strict)"("Visible"=TRUE) -> ()  [unwired: 2 in, 2 out]
                n184 = property on="Slider" class="Slide (strict)"("Visible"=FALSE) -> ()  [unwired: 2 in, 2 out]
              }
              frame Default {
                n185 = property on="Ring" class="Ring (strict)"("Visible"=FALSE) -> ()  [unwired: 2 in, 2 out]
                n186 = property on="Slider" class="Slide (strict)"("Visible"=FALSE) -> ()  [unwired: 2 in, 2 out]
              }
              frame "Brightness  **", "Color Level  **", "Compression  **", "FPS  **", "Sharpness  **" {
                n187 = call <vilib>:"NT Read Number.vi"("Name"=w316) -> ("Numeric"=w315:dbl)  [unwired: 9 in, 1 out]
                n188 = local write "Slider"(w315) -> ()
                n189 = property on="Slider" class="Slide (strict)"("Visible"=TRUE, "Scale.Maximum"=100.0 ("Scale.Range:Maximum")) -> ()  [unwired: 2 in, 2 out]
                n190 = property on="Ring" class="Ring (strict)"("Visible"=FALSE) -> ()  [unwired: 2 in, 2 out]
              }
            }
          }
        }
        n191 = property on="Progress" class="Clust (strict)"("Visible"=FALSE) -> ()  [unwired: 2 in, 2 out]
      }
      event "Test Name": Mouse Enter {
        # "Populate the ring with the list of tests"
        n192 = event-data() -> ()  [unwired: 1 in, 1 out]
        n193 = call <vilib>:"NT Read String Array.vi"("Name"="TestMode/TestList") -> ("String Array"=w323:string[])  [unwired: 9 in, 1 out]
        n194 = Build Array (concatenate)("Select the test to run...", w323) -> (w322:string[])
        n195 = property on="Test Name" class="Ring (strict)"("Strings []"=w322) -> ()  [unwired: 2 in, 2 out]
      }
      event "Test Name": Value Change {
        w325 = FALSE ("Visible")
        # "Tell the robot the test name to run"
        n196 = event-data() -> ("NewVal"=w329:u16)  [unwired: 1 in]
        n197 = property on="Test Name" class="Ring (strict)"() -> ("Strings []"=w330:string[])  [unwired: 2 in, 2 out]
        n198 = local write "Progress"(T5 {"Test Progress"=0, "Test Progress Text"=""} ("Progress")) -> ()
        n199 = Index Array(array=w330, index=w329) -> (element=w328:string)
        n200 = call <vilib>:"NT Write String.vi"("String"=w328, "Name"="TestMode/TestName") -> ()  [unwired: 9 in, 1 out]
        n201 = property on="Progress" class="Clust (strict)"("Visible"=TRUE) -> ()  [unwired: 2 in, 2 out]
        n202 = property on="Motor" class="Clust (strict)"("Visible"=w325) -> ()  [unwired: 2 in, 2 out]
        n203 = property on="Slider" class="Slide (strict)"("Visible"=w325) -> ()  [unwired: 2 in, 2 out]
        n204 = property on="On/Off" class="Bool (strict)"("Visible"=w325) -> ()  [unwired: 2 in, 2 out]
        n205 = property on="Rev/Fwd" class="Clust (strict)"("Visible"=w325) -> ()  [unwired: 2 in, 2 out]
        n206 = property on="Ring" class="Ring (strict)"("Visible"=w325) -> ()  [unwired: 2 in, 2 out]
      }
      event "Listbox": Double Click {
        n207 = event-data() -> ("PlatMods.Shift"=w333:bool, "Row"=w335:i32)  [unwired: 1 in]
        n208 = case shown="False" w333 {
          tunnel: w335 -> [w339 _]
          tunnel: 1 -> [w338 _]
          frame False {
            n209 = property on="Listbox" class="LstBox (strict)"() -> ("Item Symbols"=w337:i32[])  [unwired: 2 in, 2 out]
            n210 = Replace Array Subset(array=w337, new element=w338, index=w339) -> (w336:i32[])
            n211 = property on="Listbox" class="LstBox (strict)"("Item Symbols"=w336) -> ()  [unwired: 2 in, 2 out]
          }
          frame True {
            w340 = 0 ("Top Row")
            n212 = property on="Listbox" class="LstBox (strict)"() -> ("Number of Rows"=w342:u32)  [unwired: 2 in, 2 out]
            n213 = Initialize Array(0, w342) -> (w341:i32[])
            n214 = property on="Listbox" class="LstBox (strict)"("Top Row"=w340, "Value"=w340, "Item Symbols"=w341) -> ()  [unwired: 2 in, 2 out]
          }
        }
      }
      event "Listbox": Key Down {
        n215 = event-data() -> ("VKey"=w346:T17)  [unwired: 1 in]
        n216 = case shown="\"Left\", \"Right\"" w346 {
          selector: w346 -> [w351 _]
          tunnel: eventvkey."Left" ("VKey") -> [w349 _]
          frame "Left", "Right" {
            n217 = Equal?(x=w349, y=w351) -> (x = y?=w350:bool)
            n218 = Select(t=0, s=w350, f=1) -> (s? t:f=w352:i32)
            n219 = property on="Listbox" class="LstBox (strict)"() -> ("Item Symbols"=w355:i32[])  [unwired: 2 in, 2 out]
            n220 = Replace Array Subset(array=w355, new element=w352, index="Listbox") -> (w354:i32[])
            n221 = property on="Listbox" class="LstBox (strict)"("Item Symbols"=w354) -> ()  [unwired: 2 in, 2 out]
          }
          frame Default {
          }
        }
      }
      event "DB Camera Config": Value Change {
        n222 = event-data() -> ("NewVal"=w359:bool)  [unwired: 1 in]
        n223 = case shown="False" w359 {
          tunnel: w358 -> [w368 _]
          tunnel: [w361 w379] -> w357
          tunnel: w356 -> [w360 w379]
          frame False {
            w375 = "Camera"
            w378 = FALSE ("Visible")
            n224 = local read "Camera Settings"() -> (w367:T2)
            n225 = Index Array(array=w368) -> (element=w371:cluster{string[]})  [unwired: 1 in]
            n226 = Unbundle(w367) -> ("Frate Rate"=w366:i32, "Compression"=w365:i32, "Size"=w369:u16)
            n227 = Unbundle(w371) -> (w370:string[])
            n228 = Index Array(array=w370, index=w369) -> (element=w364:string)
            n229 = call-poly <vilib>:"Write Key.vi"("section"=w375, "value"=w364, "key"="Size", "refnum"=w360) -> ("refnum out"=w377:T16)  [unwired: 2 in, 5 out]
            n230 = call-poly <vilib>:"Write Key.vi"("section"=w375, "value"=w366, "key"="FrameRate", "refnum"=w377) -> ("refnum out"=w376:T16)  [unwired: 1 in, 6 out]
            n231 = property on="Camera Settings" class="Clust (strict)"("Visible"=w378) -> ()  [unwired: 2 in, 2 out]
            n232 = local write "DB Camera Config"(w378) -> ()
            n233 = call-poly <vilib>:"Write Key.vi"("section"=w375, "value"=w365, "key"="Compression", "refnum"=w376) -> ("refnum out"=w362:T16)  [unwired: 1 in, 6 out]
            n234 = call <vilib>:"Close Config Data.vi"("refnum"=w362) -> ("file path"=w363:path)  [unwired: 2 in, 8 out]
            n235 = call <vilib>:"Open Config Data.vi"("configuration file path"=w363) -> ("refnum"=w361:T16)  [unwired: 8 in, 2 out]
          }
          frame True {
            n236 = property on="Camera Settings" class="Clust (strict)"("Visible"=TRUE) -> ()  [unwired: 2 in, 2 out]
          }
        }
      }
      event "Camera Settings": Value Change {
        n237 = event-data() -> ("NewVal"=w392:T2)  [unwired: 1 in]
        n238 = Index Array(array=w388) -> (element=w387:cluster{string[]})  [unwired: 1 in]
        n239 = Unbundle(w392) -> ("Frate Rate"=w383:i32, "Compression"=w382:i32, "Size"=w385:u16)
        n240 = Unbundle(w387) -> (w386:string[])
        n241 = Index Array(array=w386, index=w385) -> (element=w384:string)
        n242 = Format Into String(format string="%s   %dfps   %d%%", w384, w383, w382) -> (resulting string=w389:string)  [unwired: 2 in, 1 out]
        n243 = Build Array(w389) -> (w390:string[])
        n244 = property on="DB Camera Config" class="Bool (strict)"("Strings [4]"=w390) -> ()  [unwired: 2 in, 2 out]
      }
      event "Motor.Enable": Value Change {
        n245 = event-data() -> ("NewVal"=w398:bool)  [unwired: 1 in]
        n246 = Unbundle("Motor") -> ("Value"=w397:dbl)  [unwired: 1 out]
        n247 = Select(t=w397, s=w398, f=0.0) -> (s? t:f=w395:dbl)
        n248 = call <vilib>:"NT Write Number.vi"("Numeric"=w395, "Name"=w394) -> ()  [unwired: 9 in, 1 out]
      }
      event "Slider": Value Change {
        n249 = event-data() -> ("NewVal"=w401:dbl)  [unwired: 1 in]
        n250 = call <vilib>:"NT Write Number.vi"("Numeric"=w401, "Name"=w402) -> ()  [unwired: 9 in, 1 out]
      }
      event "On/Off": Value Change {
        n251 = event-data() -> ("NewVal"=w406:bool)  [unwired: 1 in]
        n252 = Boolean To (0,1)(Boolean=w406) -> (0, 1=w405:i16)
        n253 = call <vilib>:"NT Write Number.vi"("Numeric"=w405, "Name"=w404) -> ()  [unwired: 9 in, 1 out]
      }
      event "Rev/Fwd": Value Change {
        n254 = event-data() -> ("NewVal.Forward"=w414:bool, "NewVal.Reverse"=w413:bool)  [unwired: 1 in]
        n255 = Boolean To (0,1)(Boolean=w414) -> (0, 1=w410:i16)
        n256 = Boolean To (0,1)(Boolean=w413) -> (0, 1=w412:i16)
        n257 = Negate(x=w412) -> (-x=w411:i16)
        n258 = Add(x=w410, y=w411) -> (x+y=w409:i16)
        n259 = call <vilib>:"NT Write Number.vi"("Numeric"=w409, "Name"=w408) -> ()  [unwired: 9 in, 1 out]
      }
      event "Ring": Value Change {
        n260 = event-data() -> ("NewVal"=w418:u16)  [unwired: 1 in]
        n261 = property on="Ring" class="Ring (strict)"() -> ("Strings []"=w419:string[])  [unwired: 2 in, 2 out]
        n262 = Index Array(array=w419, index=w418) -> (element=w417:string)
        n263 = call <vilib>:"NT Write String.vi"("String"=w417, "Name"=w416) -> ()  [unwired: 9 in, 1 out]
      }
    }
  }
  n264 = Index Array(array=w13) -> (element=w14:cluster{string[]})  [unwired: 1 in]
  n265 = Unbundle(w14) -> (w12:string[])
  n266 = Match First String(2:w12, 3:w11) -> (0:w10:i32)  [unwired: 1 out]
  n267 = Bundle("value"=w16, "value"=w15, "index"=w10) -> (w4:cluster{"value":i32, "value":i32, "index":i32})  [unwired: 1 out]
  n268 = property on="On/Off" class="Bool (strict)"("Visible"=w27) -> ()  [unwired: 2 in, 2 out]
  n269 = property on="Motor" class="Clust (strict)"("Visible"=w27) -> ()  [unwired: 2 in, 2 out]
  n270 = property on="Progress" class="Clust (strict)"("Visible"=w27) -> ()  [unwired: 2 in, 2 out]
  n271 = property on="Ring" class="Ring (strict)"("Visible"=w27) -> ()  [unwired: 2 in, 2 out]
  n272 = property on="Rev/Fwd" class="Clust (strict)"("Visible"=w27) -> ()  [unwired: 2 in, 2 out]
  n273 = property on="Camera Settings" class="Clust (strict)"("Val(Sgnl)"=w4) -> ()  [unwired: 2 in, 2 out]
  n274 = property on="Camera Settings" class="Clust (strict)"("Visible"=w27) -> ()  [unwired: 2 in, 2 out]
  n275 = local write "DB Camera Config"(w27) -> ()
